vi "1.3.3-Lidar Read Write.vi"   [LabVIEW 2010]
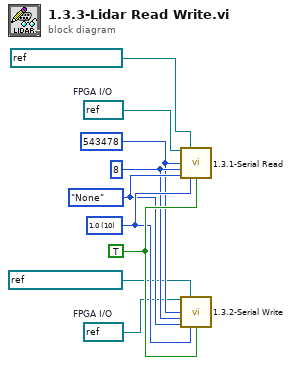
[diagram p0: block diagram]
diagram:
  w1 = refnum<k21> "Rx"  # FPGA I/O
  w2 = refnum<k21> "Tx"  # FPGA I/O
  w9 = TRUE ("Invert Polarity?")
  w8 = u16 10 items=["1.0"=10, "1.5"=15, "2.0"=20] ("stop bits (10: 1 bit)")
  w7 = enum16{"None", "Odd", "Even", "Mark", "Space"}."None" ("parity (0:none)")
  w6 = 8 ("data bits (8)")
  w5 = u32 543478 ("baud rate (9600)")
  n1 = call "1.3.1-Serial Read.vi"("Rx FPGA I/O"=w1, "Read FIFO"=refnum<k21> "2.3.2-Lidar Read", "baud rate (9600)"=w5, "data bits (8)"=w6, "parity (0:none)"=w7, "stop bits (10: 1 bit)"=w8, "Invert Polarity?"=w9) -> ()  [unwired: 9 in]
  n2 = call "1.3.2-Serial Write.vi"("Tx FPGA I/O"=w2, "Write FIFO"=refnum<k21> "2.3.1-Lidar Write", "baud rate (9600)"=w5, "data bits (8)"=w6, "parity (0:none)"=w7, "stop bits (10: 1 bit)"=w8, "Invert Polarity?"=w9) -> ()  [unwired: 9 in]
